vi "SQL Execute.vi"(8 "error in (no error)":errorcluster, 10 "Command Text":string, 11 "NI_DB_API in":refnum<class "NI_DB_API.lvclass">) -> (0 "error out":errorcluster, 1 "FirstRow":string[](array[string]), 2 "Datas":string[][](table), 3 "NI_DB_API out":refnum<class "NI_DB_API.lvclass">, 4 "Rows Fetched":i32)   [LabVIEW 2021, in "NI_DB_API.lvclass"]
uses:
  <userlib>/John_Lib/DataBase/NI_DB_API/NI_DB_API.lvclass
  <userlib>/John_Lib/DataBase/NI_DB_API/NI_DB_API.lvclass/NI_DB_API.ctl
  <vilib>/addons/database/NI_Database_API.lvlib
  <vilib>/addons/database/Connection.llb/Conn Execute.vi
  <vilib>/addons/database/Recordset.llb/Rec Destroy - Connection.vi
  <vilib>/addons/database/Recordset.llb/Rec Fetch Recordset Data (R).vi
  <userlib>/John_Lib/DataBase/DataBase_SQL/DataBase_SQL.lvclass
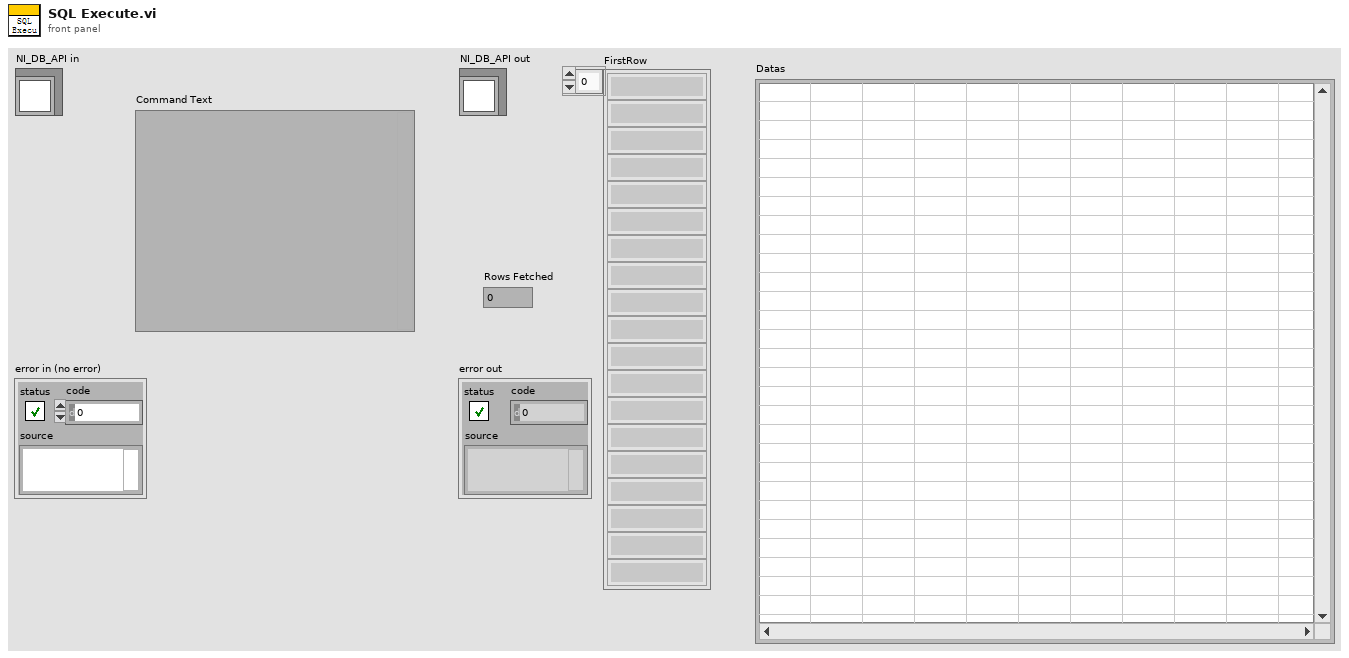
[diagram p1: front panel]
types:
  T1 = typedef "NI_Database_API.lvlib/Conn ObjectReference.ctl" = refnum<k1>
  T2 = typedef "NI_Database_API.lvlib/Rec ObjectReference.ctl" = refnum<k1>
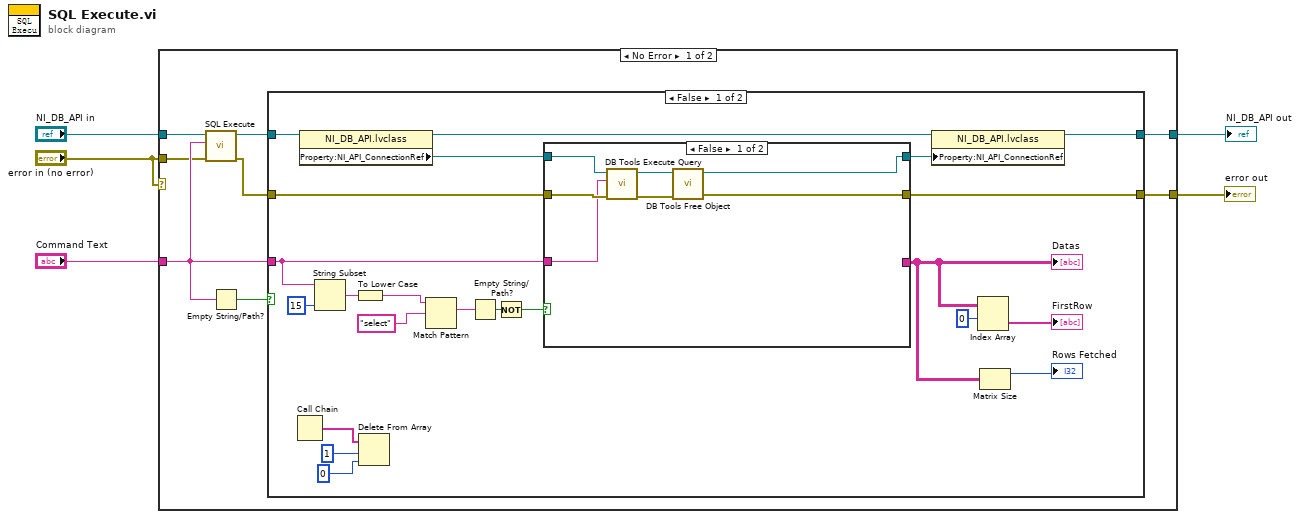
[diagram p0: block diagram]
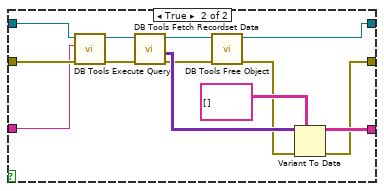
[diagram p2: hidden frame]
diagram:
  n1 = case shown="No Error" "error in (no error)" {
    selector: "error in (no error)" -> [_ w58]
    tunnel: [w12 w59] -> w5
    tunnel: [w11 w58] -> w4
    tunnel: "Command Text" -> [w10 _]
    tunnel: "NI_DB_API in" -> [w9 w59]
    tunnel: "error in (no error)" -> [w7 _]
    frame No Error {
      n2 = call-parent "SQL Execute.vi"("error in (no error)"=w7, "Command Text"=w10, "DataBase_SQL in"=w9) -> ("error out"=w6:errorcluster, "DataBase_SQL out"=w8:refnum<class "NI_DB_API.lvclass">)  [unwired: 4 in, 3 out]
      n3 = Empty String/Path?(string/path=w10) -> (empty?=w13:bool)
      n4 = case shown="False" w13 {
        tunnel: w6 -> [w35 w56]
        tunnel: [w19 w56] -> w11
        tunnel: w8 -> [w24 w57]
        tunnel: [w21 w57] -> w12
        tunnel: w10 -> [w18 _]
        frame False {
          n5 = Call Chain() -> (call chain=w28:string[])
          n6 = property class="NI_DB_API.lvclass"(reference=w24) -> (reference out=w23:refnum<class "NI_DB_API.lvclass">, "Property:NI_API_ConnectionRef"=w22:T1)  [unwired: 1 in, 1 out]
          n7 = String Subset(string=w18, length (rest)=15 ("length (rest)")) -> (substring=w26:string)  [unwired: 1 in]
          n8 = To Lower Case(string=w26) -> (all lower case string=w25:string)
          n9 = Delete From Array(array=w28, length=1, index=0) -> ()  [unwired: 2 out]
          n10 = Match Pattern(string=w25, regular expression="select") -> (match substring=w33:string)  [unwired: 1 in, 3 out]
          n11 = Empty String/Path?(string/path=w33) -> (empty?=w32:bool)
          n12 = Not(x=w32) -> (.not. x?=w31:bool)
          n13 = case shown="False" w31 {
            tunnel: w18 -> [w36 w48]
            tunnel: w35 -> [w37 w49]
            tunnel: [w38 w43] -> w19
            tunnel: w22 -> [w40 w51]
            tunnel: [w39 w50] -> w20
            tunnel: [_ w45] -> w15
            frame False {
              n14 = call-poly <vilib>:"DB Tools Execute Query.vi"("error in (no error)"=w37, "SQL query"=w36, "connection reference"=w40) -> ("error out"=w41:errorcluster, "recordset reference"=w42:T2)  [unwired: 5 in]
              n15 = call-poly <vilib>:"DB Tools Free Object.vi"("error in (no error)"=w41, "recordset reference"=w42) -> ("error out"=w38:errorcluster, "connection reference"=w39:T1)  [unwired: 8 in]
            }
            frame True {
              n16 = call-poly <vilib>:"DB Tools Execute Query.vi"("error in (no error)"=w49, "SQL query"=w48, "connection reference"=w51) -> ("error out"=w47:errorcluster, "recordset reference"=w55:T2)  [unwired: 5 in]
              n17 = call-poly <vilib>:"DB Tools Fetch Recordset Data.vi"("error in (no error)"=w47, "recordset reference"=w55) -> ("error out"=w46:errorcluster, "recordset data"=w53:variant[][], "recordset reference out"=w54:T2)  [unwired: 3 in]
              n18 = call-poly <vilib>:"DB Tools Free Object.vi"("error in (no error)"=w46, "recordset reference"=w54) -> ("error out"=w44:errorcluster, "connection reference"=w50:T1)  [unwired: 8 in]
              n19 = Variant To Data(error in=w44, type=string[][] [] ("array"), Variant=w53) -> (data=w45:string[][], error out=w43:errorcluster)
            }
          }
          "Datas" <- w15
          n20 = property class="NI_DB_API.lvclass"(reference=w23, "Property:NI_API_ConnectionRef"=w20) -> (reference out=w21:refnum<class "NI_DB_API.lvclass">)  [unwired: 1 in, 1 out]
          n21 = Index Array(array=w15, index (row)=0) -> (element=→"FirstRow":string[])  [unwired: 1 in]
          n22 = Matrix Size(0:w15) -> (1:→"Rows Fetched":i32)  [unwired: 1 out]
        }
        frame True {
        }
      }
    }
    frame Error {
    }
  }
  "error out" <- w4
  "NI_DB_API out" <- w5
